vi "Undistort Image (Greyscale).vi"(4 "Crop to Valid Pixels? (Default: True)":bool=TRUE, 5 "Border Type (Default: Constant)":T1, 6 "Use Fixed Point Remapping (Default: False)":bool, 7 "Value (Default: 0)":u8, 8 "error in (no error)":errorcluster, 9 "Greyscale Image Destination in":T2, 10 "Greyscale Image Source in":T2, 11 "Image Undistorter in":refnum<class "Image Undistorter.lvclass">) -> (0 "error out":errorcluster, 2 "Greyscale Image Destination":T2, 3 "Image Undistorter":refnum<class "Image Undistorter.lvclass">)   [LabVIEW 2020, in "image.lvlib" / "Image Undistorter.lvclass"]
doc: "Undistort the Source Image. The Destination image will be sized to fit."
uses:
  Image Undistorter.lvclass
  Greyscale Image.ctl
  Border Type.ctl
  Image Undistorter.lvclass/Image Undistorter.ctl
  ccc224f2-fea8-4097-85c8-c2b3fe04188f.vi
  <vilib>/Utility/error.llb/Error Cluster From Error Code.vi
  image.lvlib
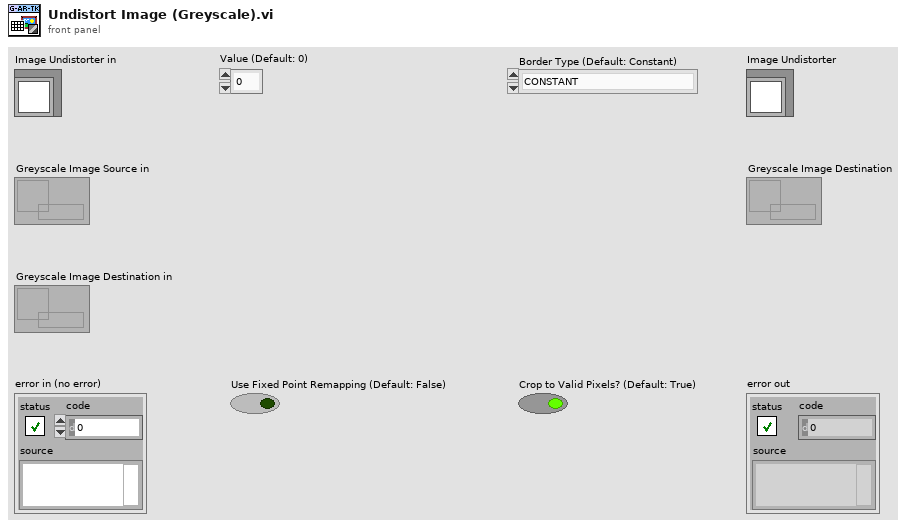
[diagram p1: front panel]
types:
  T1 = typedef "image.lvlib/Border Type.ctl" = enum8{"CONSTANT", "REPLICATE", "REFLECT", "WRAP", "TRANSPARENT", "DEFAULT", "ISOLATED"}
  T2 = typedef "image.lvlib/Greyscale Image.ctl" = refnum<data-value>
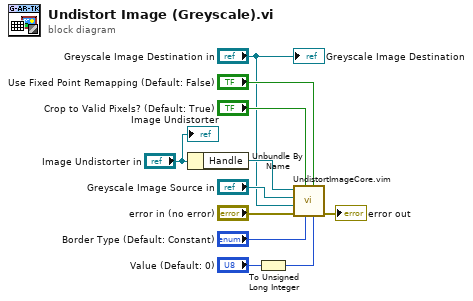
[diagram p0: block diagram]
diagram:
  n1 = Unbundle By Name("Image Undistorter in") -> ("Handle"=w10:refnum<data-value>)
  n2 = To Unsigned Long Integer(number="Value (Default: 0)") -> (unsigned 32bit integer=w1:u32)
  n3 = call "UndistortImageCore.vim"("Colour"=w1, "Use Fixed Point remapping"="Use Fixed Point Remapping (Default: False)", "Border Type"="Border Type (Default: Constant)", "Crop to Valid"="Crop to Valid Pixels? (Default: True)", "error in (no error)"="error in (no error)", "Destination Image"="Greyscale Image Destination in", "Source Image"="Greyscale Image Source in", "Handle"=w10) -> ("error out"=→"error out":errorcluster)  [unwired: 3 in]
  "Image Undistorter" <- "Image Undistorter in"
  "Greyscale Image Destination" <- "Greyscale Image Destination in"
